vi "subDFD_Allocate bits for Each Subband.vi"(10 "average bits/sample":i32=5, 11 "subband signals":waveform(dbl)[](array[waveform])) -> (2 "variance":dbl[](array[numeric]), 3 "allocated bits/sample":dbl[](array[numeric]))   [LabVIEW 2023]
uses:
  <vilib>/Analysis/NI_AALBase.lvlib
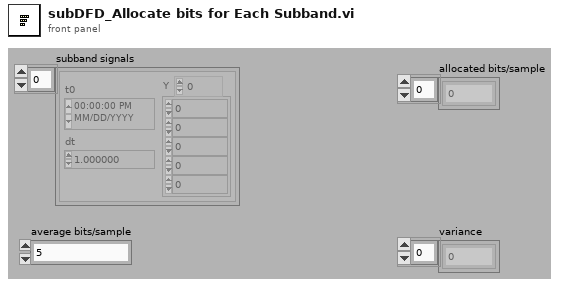
[diagram p1: front panel]
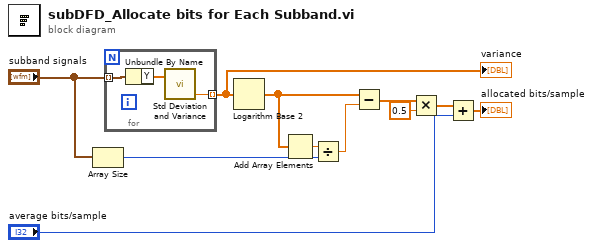
[diagram p0: block diagram]
diagram:
  n1 = Array Size(array="subband signals") -> (size(s)=w3:i32)
  n2 = for {
    tunnel: "subband signals" -> [w14] mode=indexing
    tunnel: [w13] -> w1 mode=indexing
    n3 = Unbundle By Name(w14) -> ("Y"=w12:dbl[])
    n4 = call <vilib>:"Std Deviation and Variance.vi"("X"=w12) -> ("variance"=w13:dbl)  [unwired: 1 in, 2 out]
  }
  "variance" <- w1
  n5 = Logarithm Base 2(1:w1) -> (0:w2:dbl[])
  n6 = Add Array Elements(numeric array=w2) -> (sum=w5:dbl)
  n7 = Divide(x=w5, y=w3) -> (x/y=w6:dbl)
  n8 = Subtract(x=w2, y=w6) -> (x-y=w7:dbl[])
  n9 = Multiply(x=w7, y=0.5 ("x/y")) -> (x*y=w10:dbl[])
  n10 = Add(x=w10, y="average bits/sample") -> (x+y=→"allocated bits/sample":dbl[])
